vi "ProcessFCCurrents.vi"(9 "FC Data":waveform(dbl)[](array[waveform]), 10 "Bouncer Settings":T1, 11 "FC Offset":T2) -> (1 "Mean Currents":dbl[](array[numeric]), 2 "Output Waveforms":waveform(dbl)[](array[waveform]))   [LabVIEW 2011]
uses:
  <vilib>/Waveform/WDTOps.llb/WDT Get Waveform Subset DBL (LV80).vi
  <vilib>/Analysis/NI_AALBase.lvlib
panel:
  out "HE 13CL":dbl
  out "HE 13CH":waveform(dbl)
  out "LE 13C":dbl
  out "HE 13CH":dbl
  out "LE 12C":dbl
  out "HE 12C":dbl
  out "Bouncer":waveform(dbl)(graph)={"t0"=timestamp(3415120333.4009705 s since 1904-01-01), "dt"=9.999999999999972e-06, "Y"=array[1000 elements], "attributes"=variant("NI_ChannelName"=variant(string "PXI1Slot2/ai0"), "NI_UnitDescription"=variant(string "Volts"))}
  out "LE 13C Cup":waveform(dbl)(graph)={"t0"=timestamp(3415120333.402178 s since 1904-01-01), "dt"=9.999999999999972e-06, "Y"=[0.8050097183722652, 0.24660166407635983, 0.028584441505206795, 0.009584422869030943, 0.009906457076575987, 0.00797425183471986, 0.00797425183471986, 0.007008149216862962, 0.012804764954733521, 0.01312679916455761, 0.010550525492349248, 0.010872559700577551, 0.009584422869030943, 0.01022849128434874, 0.01151662811771772, 0.010872559700577551, 0.010872559700577551, 0.010872559700577551, 0.01022849128434874, 0.009262388661713566, 0.004109841375562904, 0.009262388661713566, 0.01151662811771772, 0.01022849128434874, 0.019567483409006912, 0.01151662811771772, 0.010872559700577551, 0.009906457076575987, 0.009584422869030943, 0.01022849128434874, 0.013448833374609843, 0.01022849128434874, 0.009906457076575987, 0.010550525492349248, 0.00668611501136536, 0.010550525492349248, 0.01022849128434874, 0.01022849128434874, 0.009584422869030943, 0.013448833374609843], "attributes"=variant("NI_ChannelName"=variant(string "PXI1Slot2/ai3"), "NI_UnitDescription"=variant(string "Volts"))}
  out "LE 12C Cup":waveform(dbl)(graph)={"t0"=timestamp(3415120333.4013777 s since 1904-01-01), "dt"=9.999999999999972e-06, "Y"=[0.00668611501136536, 0.007008149216862962, 0.007652217628540168, 0.007330183422587883, 0.00861832024776164, 0.007330183422587883, 0.009262388661713566, 0.01312679916455761, 0.05338107720327494, 0.6781279926088322, 0.8175690797952145, 0.8223996035554544, 0.8240097781590372, 0.8233657083165931, 0.8249758829252316, 0.8230436733958766, 0.8243318130807649, 0.8236877432376466, 0.8243318130807649, 0.8243318130807649, 0.8233657083165931, 0.8278741972420289, 0.8236877432376466, 0.8240097781590372, 0.8227216384754971, 0.8246538480028296, 0.8246538480028296, 0.8246538480028296, 0.8249758829252316, 0.8252979178479707, 0.8214334987973474, 0.8236877432376466, 0.8246538480028296, 0.8246538480028296, 0.8227216384754971, 0.8236877432376466, 0.8243318130807649, 0.8217555337163797, 0.8240097781590372, 0.8243318130807649], "attributes"=variant("NI_ChannelName"=variant(string "PXI1Slot2/ai3"), "NI_UnitDescription"=variant(string "Volts"))}
  out "HE 13CL Cup":waveform(dbl)(graph)={"t0"=timestamp(3415120333.4017754 s since 1904-01-01), "dt"=9.999999999999972e-06, "Y"=[0.41889009921070675, 0.6410939957678486, 0.7270772818431984, 0.7261111773784867, 0.7270772818431984, 0.7293315256055366, 0.7267552470213039, 0.7286874559575331, 0.7306196649054364, 0.7254671077369653, 0.7283654211340178, 0.7302976300799747, 0.7277213514879598, 0.7261111773784867, 0.7306196649054364, 0.7341620480069433, 0.7293315256055366, 0.7302976300799747, 0.7319078042105287, 0.7331959435208164, 0.7280433863108267, 0.7331959435208164, 0.7290094907813727, 0.7299755952548376, 0.7309416997312226, 0.7344840828363023, 0.7293315256055366, 0.7299755952548376, 0.7267552470213039, 0.7338400131779094, 0.7219247247317432, 0.7225687943661443, 0.7280433863108267, 0.7280433863108267, 0.7309416997312226, 0.7290094907813727, 0.7328739086927573, 0.7277213514879598, 0.7161280980802982, 0.7286874559575331], "attributes"=variant("NI_ChannelName"=variant(string "PXI1Slot2/ai2"), "NI_UnitDescription"=variant(string "Volts"))}
  out "HE 12C Cup":waveform(dbl)(graph)={"t0"=timestamp(3415120333.400973 s since 1904-01-01), "dt"=9.999999999999972e-06, "Y"=[-0.00168677425192447, 0.003143738765882537, -0.002652876849375083, -0.00168677425192447, 0.0008894993512310448, -0.002652876849375083, 0.0005674651500443148, -0.000720671652438485, 0.0018556019561503992, 0.0018556019561503992, 0.0024996703605630385, 0.0015335677542840436, 0.002177636158243383, -0.0013647400523220184, 0.005397978191647298, 0.0018556019561503992, 0.0012115335526442733, 0.0015335677542840436, 0.016669175487689536, 0.2607711773435167, 0.6375516136789285, 0.6369075442122739, 0.6423821347186465, 0.6456024821175347, 0.6449584126352536, 0.6423821347186465, 0.6456024821175347, 0.6427041694571275, 0.639805856822051, 0.6427041694571275, 0.6388397526159826, 0.6449584126352536, 0.6423821347186465, 0.6443143431542244, 0.6452804473762376, 0.6401278915580318, 0.6410939957678486, 0.6468906210858548, 0.6446363778945825, 0.6433482389350278], "attributes"=variant("NI_ChannelName"=variant(string "PXI1Slot2/ai1"), "NI_UnitDescription"=variant(string "Volts"))}
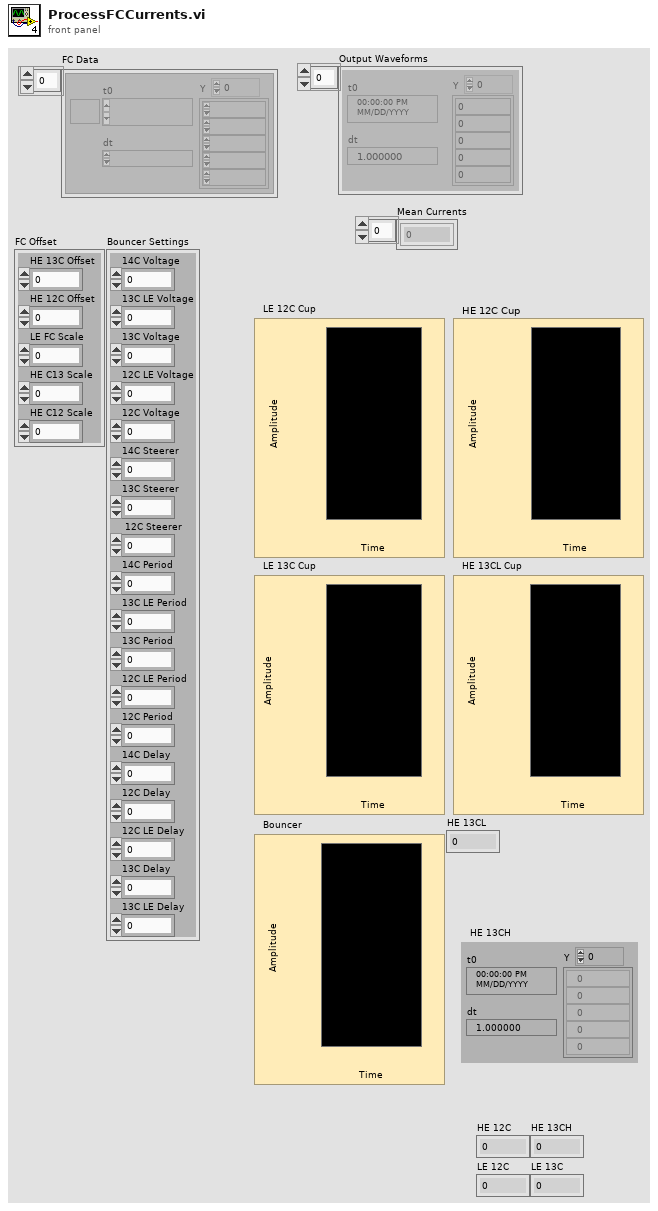
[diagram p1: front panel]
types:
  T1 = cluster{"14C Voltage":dbl, "13C LE Voltage":dbl, "13C Voltage":dbl, "12C LE Voltage":dbl, "12C Voltage":dbl, "14C Steerer":dbl, "13C Steerer":dbl, " 12C Steerer":dbl, "14C Period":dbl, "13C LE Period":dbl, "13C Period":dbl, "12C LE Period":dbl, "12C Period":dbl, "14C Delay":dbl, "12C Delay":dbl, "12C LE Delay":dbl, "13C Delay":dbl, "13C LE Delay":dbl}
  T2 = cluster{"HE 13C Offset":dbl, "HE 12C Offset":dbl, "LE FC Scale":u16, "HE C13 Scale":u16, "HE C12 Scale":u16}
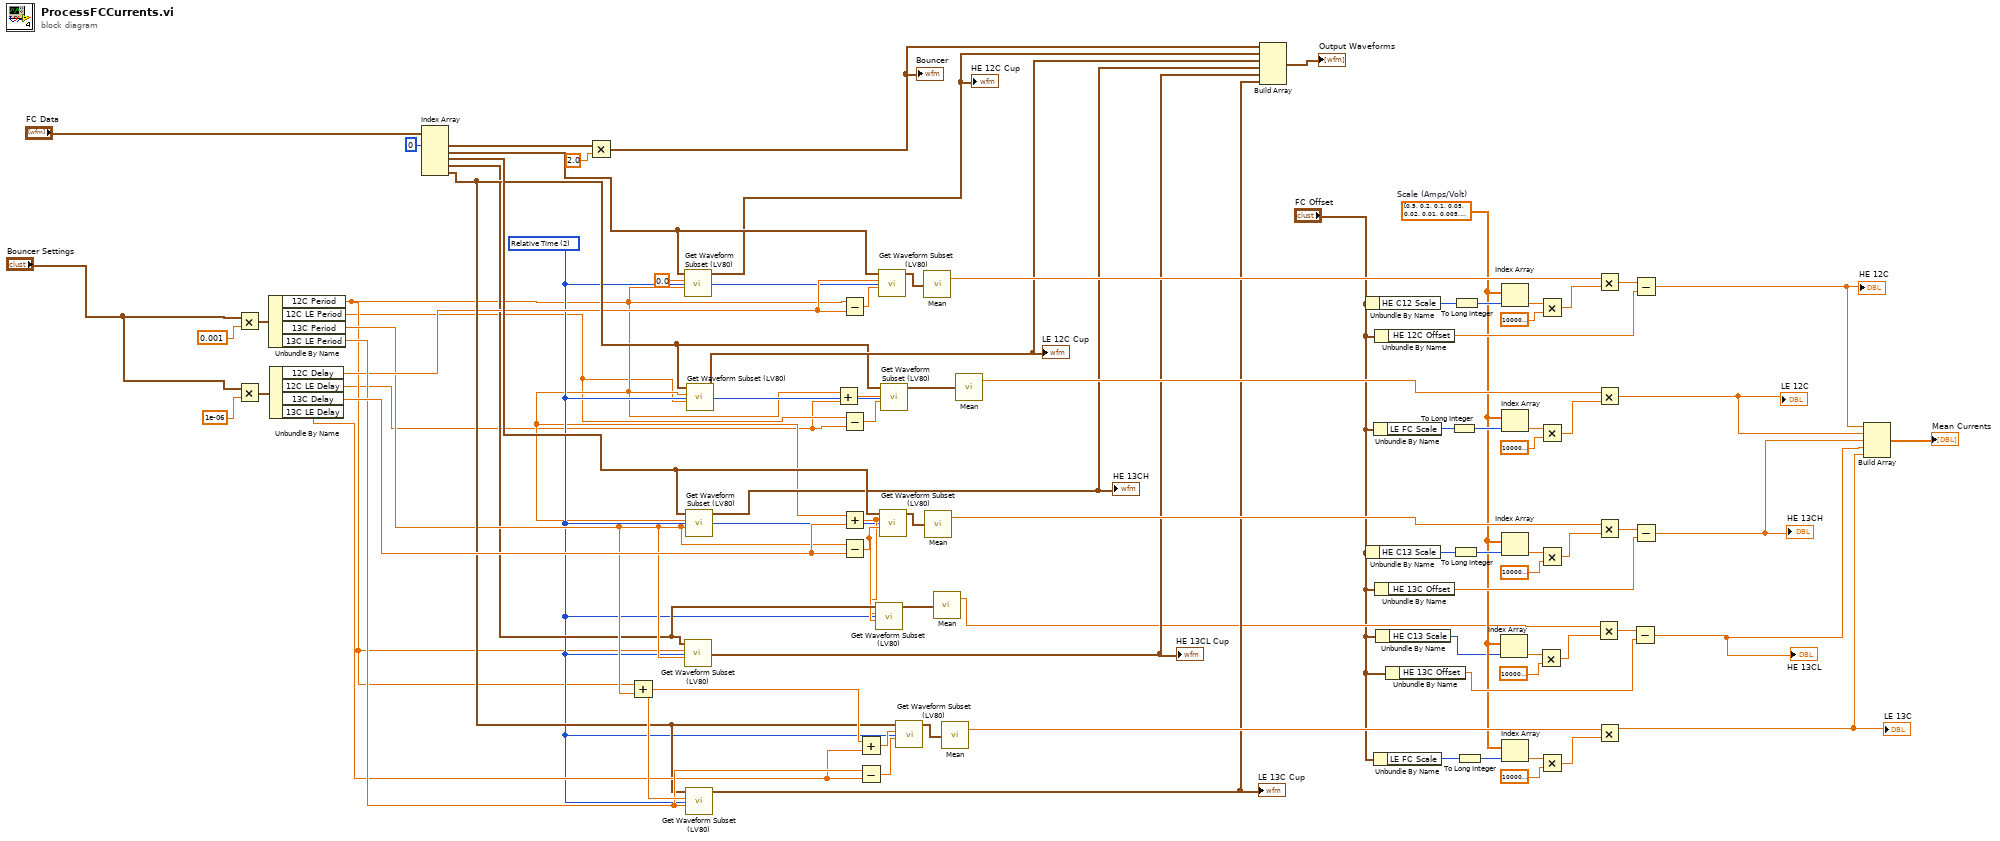
[diagram p0: block diagram]
diagram:
  w9 = dbl[] [0.5, 0.2, 0.1, 0.05, 0.02, 0.01, 0.005, 0.002, 0.001, 0.0005, 0.0002, 0.0001, 5e-05, 2e-05, 1e-05, 5e-06, 2e-06, 1e-06, 5e-07, 2e-07, 1e-07, 5e-08, 2e-08, 1e-08, 5e-09, 2e-09, 1e-09, 5e-10, 2e-10, 1e-10, 5e-11, 2e-11, 1e-11, 5e-12, 2e-12, 1e-12]  # Scale (Amps/Volt)
  w17 = u16 2 items=["Samples", "Absolute Time", "Relative Time"] ("start/duration format")
  n1 = Multiply(x="Bouncer Settings", y=0.001) -> (x*y=w83:T1)
  n2 = Multiply(x="Bouncer Settings", y=1e-06) -> (x*y=w81:T1)
  n3 = Unbundle By Name(w83) -> ("12C Period"=w5:dbl, "12C LE Period"=w2:dbl, "13C Period"=w21:dbl, "13C LE Period"=w70:dbl)
  n4 = Unbundle By Name(w81) -> ("12C Delay"=w23:dbl, "12C LE Delay"=w1:dbl, "13C Delay"=w75:dbl, "13C LE Delay"=w69:dbl)
  n5 = Index Array(array="FC Data", index #1=0 ("index")) -> (element #1=w85:waveform(dbl), element #2=w39:waveform(dbl), element #3=w38:waveform(dbl), element #4=w20:waveform(dbl), element #5=w26:waveform(dbl))  [unwired: 4 in]
  n6 = Multiply(x=w85, y=2.0) -> (x*y=w36:waveform(dbl))
  "Bouncer" <- w36
  n7 = Add(x=w5, y=w21) -> (x+y=w71:dbl)
  n8 = call-poly <vilib>:"Get Waveform Subset (LV80).vi"("start/duration format"=w17, "duration"=w5, "start samples/time"=0.0, "waveform in"=w39) -> ("waveform out"=w35:waveform(dbl))  [unwired: 1 in, 4 out]
  "HE 12C Cup" <- w35
  n9 = call-poly <vilib>:"Get Waveform Subset (LV80).vi"("start/duration format"=w17, "duration"=w21, "start samples/time"=w5, "waveform in"=w20) -> ("waveform out"=w25:waveform(dbl))  [unwired: 1 in, 4 out]
  "HE 13CL Cup" <- w25
  n10 = call-poly <vilib>:"Get Waveform Subset (LV80).vi"("start/duration format"=w17, "duration"=w21, "start samples/time"=w5, "waveform in"=w38) -> ("waveform out"=w24:waveform(dbl))  [unwired: 1 in, 4 out]
  "HE 13CH" <- w24
  n11 = call-poly <vilib>:"Get Waveform Subset (LV80).vi"("start/duration format"=w17, "duration"=w70, "start samples/time"=w71, "waveform in"=w26) -> ("waveform out"=w33:waveform(dbl))  [unwired: 1 in, 4 out]
  "LE 13C Cup" <- w33
  n12 = call-poly <vilib>:"Get Waveform Subset (LV80).vi"("start/duration format"=w17, "duration"=w2, "start samples/time"=w5, "waveform in"=w26) -> ("waveform out"=w34:waveform(dbl))  [unwired: 1 in, 4 out]
  "LE 12C Cup" <- w34
  n13 = Add(x=w5, y=w1) -> (x+y=w4:dbl)
  n14 = Subtract(x=w5, y=w23) -> (x-y=w22:dbl)
  n15 = Subtract(x=w2, y=w1) -> (x-y=w3:dbl)
  n16 = Add(x=w5, y=w75) -> (x+y=w18:dbl)
  n17 = Subtract(x=w21, y=w75) -> (x-y=w19:dbl)
  n18 = Add(x=w71, y=w69) -> (x+y=w72:dbl)
  n19 = Subtract(x=w70, y=w69) -> (x-y=w74:dbl)
  n20 = call-poly <vilib>:"Get Waveform Subset (LV80).vi"("start/duration format"=w17, "duration"=w19, "start samples/time"=w18, "waveform in"=w20) -> ("waveform out"=w16:waveform(dbl))  [unwired: 1 in, 4 out]
  n21 = call-poly <vilib>:"Get Waveform Subset (LV80).vi"("start/duration format"=w17, "duration"=w22, "start samples/time"=w23, "waveform in"=w39) -> ("waveform out"=w79:waveform(dbl))  [unwired: 1 in, 4 out]
  n22 = call-poly <vilib>:"Get Waveform Subset (LV80).vi"("start/duration format"=w17, "duration"=w19, "start samples/time"=w18, "waveform in"=w38) -> ("waveform out"=w76:waveform(dbl))  [unwired: 1 in, 4 out]
  n23 = call-poly <vilib>:"Get Waveform Subset (LV80).vi"("start/duration format"=w17, "duration"=w3, "start samples/time"=w4, "waveform in"=w26) -> ("waveform out"=w78:waveform(dbl))  [unwired: 1 in, 4 out]
  n24 = call-poly <vilib>:"Get Waveform Subset (LV80).vi"("start/duration format"=w17, "duration"=w74, "start samples/time"=w72, "waveform in"=w26) -> ("waveform out"=w73:waveform(dbl))  [unwired: 1 in, 4 out]
  n25 = call <vilib>:"Mean.vi"("X"=w79) -> ("mean"=w58:dbl)  [unwired: 1 out]
  n26 = call <vilib>:"Mean.vi"("X"=w76) -> ("mean"=w54:dbl)  [unwired: 1 out]
  n27 = call <vilib>:"Mean.vi"("X"=w16) -> ("mean"=w7:dbl)  [unwired: 1 out]
  n28 = call <vilib>:"Mean.vi"("X"=w73) -> ("mean"=w53:dbl)  [unwired: 1 out]
  n29 = call <vilib>:"Mean.vi"("X"=w78) -> ("mean"=w57:dbl)  [unwired: 1 out]
  n30 = Build Array(w36, w35, w34, w24, w25, w33) -> (→"Output Waveforms":waveform(dbl)[])
  n31 = Unbundle By Name("FC Offset") -> ("HE C12 Scale"=w68:u16)
  n32 = Unbundle By Name("FC Offset") -> ("HE C13 Scale"=w50:u16)
  n33 = Unbundle By Name("FC Offset") -> ("LE FC Scale"=w51:u16)
  n34 = Unbundle By Name("FC Offset") -> ("LE FC Scale"=w49:u16)
  n35 = Unbundle By Name("FC Offset") -> ("HE 12C Offset"=w45:dbl)
  n36 = Unbundle By Name("FC Offset") -> ("HE 13C Offset"=w46:dbl)
  n37 = Unbundle By Name("FC Offset") -> ("HE C13 Scale"=w8:u16)
  n38 = Unbundle By Name("FC Offset") -> ("HE 13C Offset"=w10:dbl)
  n39 = To Long Integer(number=w51) -> (32bit integer=w43:i32)
  n40 = To Long Integer(number=w50) -> (32bit integer=w42:i32)
  n41 = To Long Integer(number=w68) -> (32bit integer=w44:i32)
  n42 = To Long Integer(number=w49) -> (32bit integer=w41:i32)
  n43 = Index Array(array=w9, index=w8) -> (element=w15:dbl)
  n44 = Index Array(array=w9, index=w44) -> (element=w67:dbl)
  n45 = Index Array(array=w9, index=w43) -> (element=w65:dbl)
  n46 = Index Array(array=w9, index=w42) -> (element=w63:dbl)
  n47 = Index Array(array=w9, index=w41) -> (element=w61:dbl)
  n48 = Multiply(x=w15, y=1000000000.0 ("x")) -> (x*y=w13:dbl)
  n49 = Multiply(x=w67, y=1000000.0 ("x")) -> (x*y=w59:dbl)
  n50 = Multiply(x=w65, y=1000000.0 ("x")) -> (x*y=w56:dbl)
  n51 = Multiply(x=w63, y=1000000000.0 ("x")) -> (x*y=w55:dbl)
  n52 = Multiply(x=w61, y=1000000000.0 ("x")) -> (x*y=w52:dbl)
  n53 = Multiply(x=w7, y=w13) -> (x*y=w12:dbl)
  n54 = Multiply(x=w58, y=w59) -> (x*y=w48:dbl)
  n55 = Multiply(x=w57, y=w56) -> (x*y=w30:dbl)
  "LE 12C" <- w30
  n56 = Multiply(x=w54, y=w55) -> (x*y=w47:dbl)
  n57 = Multiply(x=w53, y=w52) -> (x*y=w28:dbl)
  "LE 13C" <- w28
  n58 = Subtract(x=w12, y=w10) -> (x-y=w11:dbl)
  "HE 13CL" <- w11
  n59 = Subtract(x=w48, y=w45) -> (x-y=w31:dbl)
  "HE 12C" <- w31
  n60 = Subtract(x=w47, y=w46) -> (x-y=w29:dbl)
  "HE 13CH" <- w29
  n61 = Build Array(w31, w30, w29, w11, w28) -> (→"Mean Currents":dbl[])
